vi "电池组信息解析.vi"(7 "电池组信息?":bool, 8 "Protocol_Version":dbl[](array[numeric]), 9 "BatInfor":dbl[](array[numeric]), 10 "BatDate":dbl[](array[numeric]), 11 "BatManufactorer":dbl[](array[numeric])) -> (0 "协议版本号":T1, 3 "电池信息输出":T2)   [LabVIEW 2013]
panel:
  # "电池类型:\n1:磷酸铁锂\n2:锰酸锂\n电池厂家:\n1:普莱德\n2:盟固利\n运行模式:\n1:快换\n2:非快换\n电池地区(电池应用类型)"
  # "应用类型:\n1:纯电动BMS\n2:混合动力BMS\n3:储能\n4:快换\n协议是否公开\n1:公开\n0:不公开"
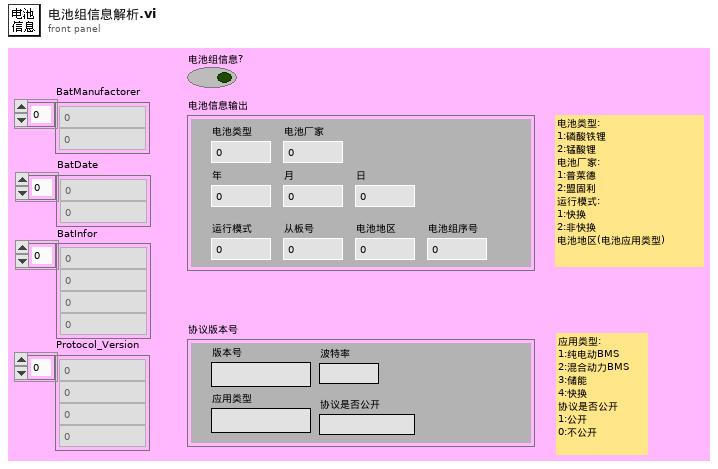
[diagram p1: front panel]
types:
  T1 = cluster{"版本号":string, "应用类型":string, "波特率":string, "协议是否公开":string}
  T2 = cluster{"电池类型":dbl, "电池厂家":dbl, "年":dbl, "月":dbl, "日":dbl, "运行模式":dbl, "从板号":dbl, "电池地区":dbl, "电池组序号":dbl}
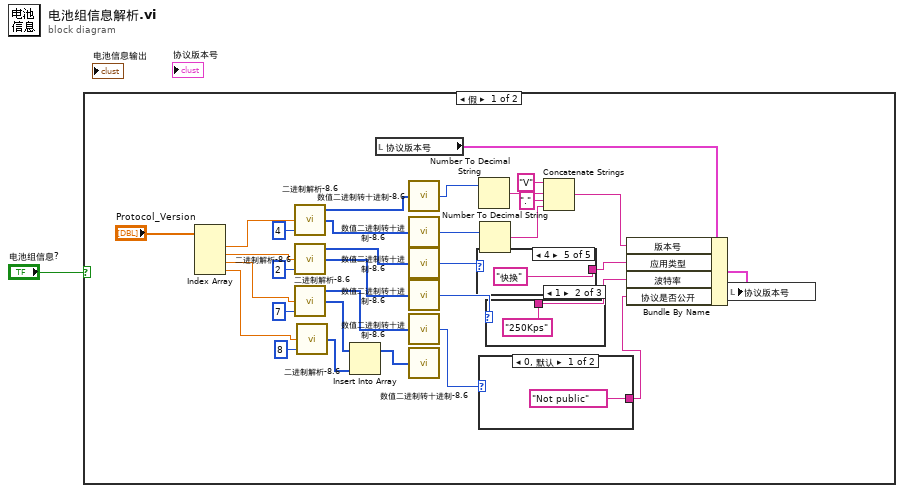
[diagram p0: block diagram]
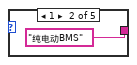
[diagram p3: hidden frame]
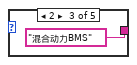
[diagram p4: hidden frame]
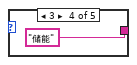
[diagram p5: hidden frame]
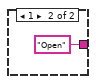
[diagram p6: hidden frame]
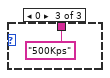
[diagram p8: hidden frame]
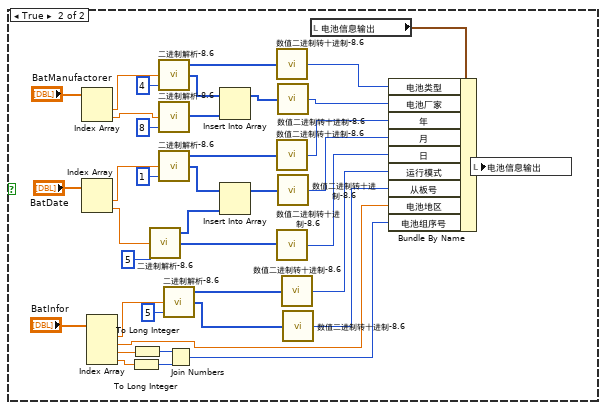
[diagram p9: hidden frame]
diagram:
  n1 = case shown="假" "电池组信息?" {
    frame False {
      n2 = Index Array(array="Protocol_Version") -> (element #1=w32:dbl, element #2=w29:dbl, element #3=w27:dbl, element #4=w26:dbl)  [unwired: 4 in]
      n3 = call "二进制解析-8.6.vi"("索引"=4, "数值"=w32) -> ("低位子数组"=w18:i32[], "高位子数组"=w17:i32[])  [unwired: 2 out]
      n4 = call "二进制解析-8.6.vi"("索引"=2, "数值"=w29) -> ("低位子数组"=w20:i32[], "高位子数组"=w19:i32[])  [unwired: 2 out]
      n5 = call "二进制解析-8.6.vi"("索引"=7, "数值"=w27) -> ("低位子数组"=w23:i32[], "高位子数组"=w21:i32[])  [unwired: 2 out]
      n6 = call "二进制解析-8.6.vi"("索引"=8, "数值"=w26) -> ("低位子数组"=w24:i32[])  [unwired: 3 out]
      n7 = Insert Into Array(array=w23, new element=w24) -> (w22:i32[])  [unwired: 1 in]
      n8 = local read "协议版本号"() -> (w16:T1)
      n9 = call "数值二进制转十进制-8.6.vi"("子数组"=w17) -> ("十进制数值"=w12:i32)  [unwired: 4 out]
      n10 = call "数值二进制转十进制-8.6.vi"("子数组"=w18) -> ("十进制数值"=w11:i32)  [unwired: 4 out]
      n11 = call "数值二进制转十进制-8.6.vi"("子数组"=w19) -> ("十进制数值"=w3:i32)  [unwired: 4 out]
      n12 = call "数值二进制转十进制-8.6.vi"("子数组"=w20) -> ("十进制数值"=w14:i32)  [unwired: 4 out]
      n13 = call "数值二进制转十进制-8.6.vi"("子数组"=w21) -> ("十进制数值"=w5:i32)  [unwired: 4 out]
      n14 = call "数值二进制转十进制-8.6.vi"("子数组"=w22) -> ()  [unwired: 5 out]
      n15 = case shown="4" w3 {
        tunnel: [_ "纯电动BMS" "混合动力BMS" "储能" "快换"] -> w2
        frame 99, Default {
        }
        frame 1 {
        }
        frame 2 {
        }
        frame 3 {
        }
        frame 4 {
        }
      }
      n16 = Number To Decimal String(number=w12) -> (decimal integer string=w10:string)  [unwired: 1 out]
      n17 = case shown="0, 默认" w5 {
        tunnel: ["Not public" "Open"] -> w4
        frame 0, Default {
        }
        frame 1 {
        }
      }
      n18 = Number To Decimal String(number=w11) -> (decimal integer string=w9:string)  [unwired: 1 out]
      n19 = case shown="1" w14 {
        tunnel: [_ "250Kps" "500Kps"] -> w13
        frame 99, Default {
        }
        frame 1 {
        }
        frame 0 {
        }
      }
      n20 = Concatenate Strings("V" ("字符串"), w10, "." ("字符串"), w9) -> (w6:string)
      n21 = Bundle By Name(cluster=w16, "版本号"=w6, "应用类型"=w2, "波特率"=w13, "协议是否公开"=w4) -> (w15:T1)
      n22 = local write "协议版本号"(w15) -> ()
    }
    frame True {
      n23 = Index Array(array="BatManufactorer") -> (element #1=w79:dbl, element #2=w76:dbl)  [unwired: 2 in]
      n24 = Index Array(array="BatDate") -> (element #1=w61:dbl, element #2=w64:dbl)  [unwired: 2 in]
      n25 = Index Array(array="BatInfor") -> (element #1=w54:dbl, element #2=w43:dbl, element #3=w50:dbl, element #4=w49:dbl)  [unwired: 4 in]
      n26 = To Long Integer(number=w49) -> (32bit integer=w47:i32)
      n27 = To Long Integer(number=w50) -> (32bit integer=w48:i32)
      n28 = call "二进制解析-8.6.vi"("索引"=5, "数值"=w64) -> ("低位子数组"=w58:i32[], "高位子数组"=w59:i32[])  [unwired: 2 out]
      n29 = call "二进制解析-8.6.vi"("索引"=4, "数值"=w79) -> ("低位子数组"=w75:i32[], "高位子数组"=w72:i32[])  [unwired: 2 out]
      n30 = call "二进制解析-8.6.vi"("索引"=8, "数值"=w76) -> ("低位子数组"=w74:i32[])  [unwired: 3 out]
      n31 = call "二进制解析-8.6.vi"("索引"=1, "数值"=w61) -> ("低位子数组"=w65:i32[], "高位子数组"=w67:i32[])  [unwired: 2 out]
      n32 = call "二进制解析-8.6.vi"("索引"=5, "数值"=w54) -> ("低位子数组"=w46:i32[], "高位子数组"=w52:i32[])  [unwired: 2 out]
      n33 = Join Numbers(hi=w48, lo=w47) -> ((hi.lo)=w42:u64)
      n34 = Insert Into Array(array=w75, new element=w74) -> (w73:i32[])  [unwired: 1 in]
      n35 = Insert Into Array(array=w65, new element=w59) -> (w66:i32[])  [unwired: 1 in]
      n36 = call "数值二进制转十进制-8.6.vi"("子数组"=w72) -> ("十进制数值"=w69:i32)  [unwired: 4 out]
      n37 = call "数值二进制转十进制-8.6.vi"("子数组"=w67) -> ("十进制数值"=w57:i32)  [unwired: 4 out]
      n38 = call "数值二进制转十进制-8.6.vi"("子数组"=w58) -> ("十进制数值"=w55:i32)  [unwired: 4 out]
      n39 = call "数值二进制转十进制-8.6.vi"("子数组"=w73) -> ("十进制数值"=w68:i32)  [unwired: 4 out]
      n40 = call "数值二进制转十进制-8.6.vi"("子数组"=w66) -> ("十进制数值"=w56:i32)  [unwired: 4 out]
      n41 = call "数值二进制转十进制-8.6.vi"("子数组"=w52) -> ("十进制数值"=w45:i32)  [unwired: 4 out]
      n42 = call "数值二进制转十进制-8.6.vi"("子数组"=w46) -> ("十进制数值"=w44:i32)  [unwired: 4 out]
      n43 = local read "电池信息输出"() -> (w70:T2)
      n44 = Bundle By Name(cluster=w70, "电池类型"=w69, "电池厂家"=w68, "年"=w57, "月"=w56, "日"=w55, "运行模式"=w45, "从板号"=w44, "电池地区"=w43, "电池组序号"=w42) -> (w71:T2)
      n45 = local write "电池信息输出"(w71) -> ()
    }
  }
